vi "Main.vi"() -> ()   [LabVIEW 2014]
uses:
  <vilib>/addons/Fuzzy Logic/NI_Fuzzy_Logic_API.lvlib
  <vilib>/addons/Fuzzy Logic/FL Fuzzy Controller (MISO).vi
  <vilib>/express/express arith-compare/Formula/XNode/ExpressFormulaBlockNode.xnode
  <vilib>/express/express shared/transition.llb/Dynamic To Waveform Array.vi
  <vilib>/express/express arith-compare/Formula/Block/exnFormulaBlock how many pts in the wave.vi
  <vilib>/express/express shared/ex_Modify Signal Name.vi
  <vilib>/express/express shared/transition.llb/Waveform Array To Dynamic.vi
panel:
  out "Control History":dbl(graph)
  out "Sensors History":dynamicdata(graph)
  out "Error bar":string
  out "Information":string
  out "Danger":bool
  out "Status":string
  out "Thermistor III":dbl(slide) scale=0.0..100.0
  out "Thermistor II":dbl(slide) scale=0.0..100.0
  out "LM-35 II":dbl(slide) scale=0.0..100.0
  out "LM-35 III":dbl(slide) scale=0.0..100.0
  out "Thermistor I":dbl(slide) scale=0.0..100.0
  out "LM-35 I":dbl(slide) scale=0.0..100.0
  out "Final Control":dbl(knob) scale=0.0..1.0
  out "LM-35 Intel":dbl(knob) scale=0.0..10.0
  out "Thermistors Intel":dbl(knob) scale=0.0..10.0
  in  "Control System":bool
  # "In Celsius"
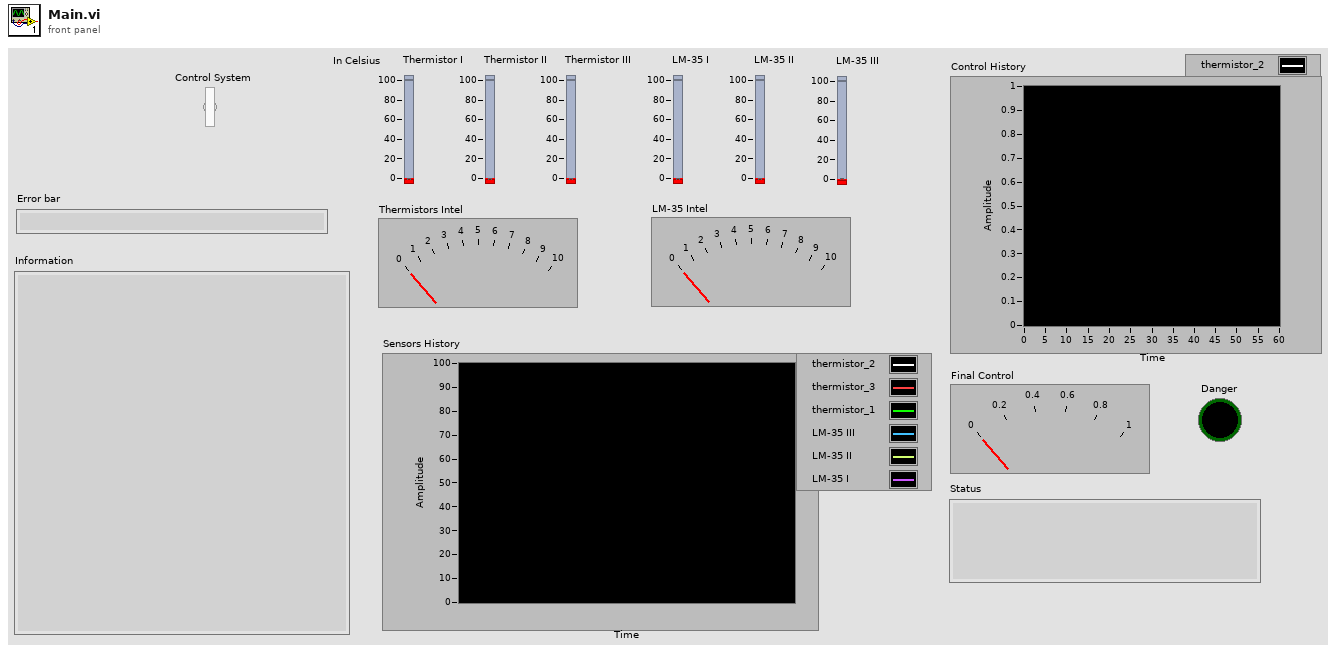
[diagram p1: front panel]
types:
  T1 = typedef "NI_Fuzzy_Logic_API.lvlib/FL System.ctl" = cluster{"input variables":T2[], "output variables":T2[], "rules":T5[], "defuzzification method":T11, "description":string, "user MF interpolating polynomials":T12[]}
  T2 = typedef "NI_Fuzzy_Logic_API.lvlib/FL Variable.ctl" = cluster{"name":string, "range":dbl[], "MFs":T3[]}
  T3 = typedef "NI_Fuzzy_Logic_API.lvlib/FL Membership Function.ctl" = cluster{"name":string, "shape":T4, "points":dbl[], "color":u32, "user-defined shape index":i32}
  T4 = typedef "NI_Fuzzy_Logic_API.lvlib/FL Membership Function Shape.ctl" = u16
  T5 = typedef "NI_Fuzzy_Logic_API.lvlib/FL Rule.ctl" = cluster{"antecedents":T6[], "antecedent connective":T8, "consequents":T9[], "consequent implication":T10, "degree of support":dbl}
  T6 = typedef "NI_Fuzzy_Logic_API.lvlib/FL Antecedent.ctl" = cluster{"Var Index":i32, "MF Index":i32, "Cond":T7}
  T7 = typedef "NI_Fuzzy_Logic_API.lvlib/FL Modifier.ctl" = u16
  T8 = typedef "NI_Fuzzy_Logic_API.lvlib/FL Antecedent Connective.ctl" = u16
  T9 = typedef "NI_Fuzzy_Logic_API.lvlib/FL Consequent.ctl" = cluster{"Var Index":i32, "MF Index":i32, "Cond":T7}
  T10 = typedef "NI_Fuzzy_Logic_API.lvlib/FL Consequent Implication.ctl" = u16
  T11 = typedef "NI_Fuzzy_Logic_API.lvlib/FL Defuzzification.ctl" = u16
  T12 = typedef "NI_Fuzzy_Logic_API.lvlib/FL Interpolating polynomials.ctl" = cluster{"X":dbl[], "Y":dbl[], "Y(x) coeff":dbl[][], "X(y) coeff":dbl[][], "Area(y) coeff":dbl[][], "coa_x(y) coeff":dbl[][]}
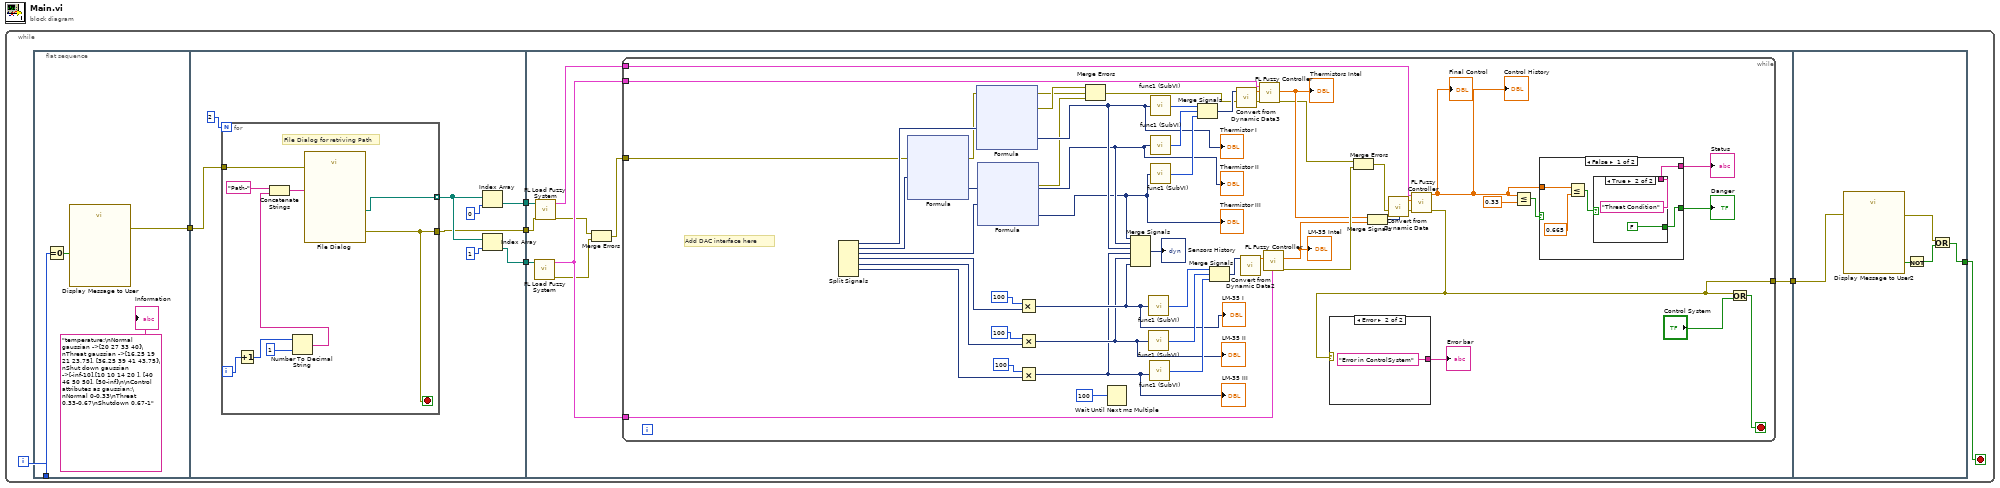
[diagram p0: block diagram]
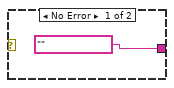
[diagram p2: hidden frame]
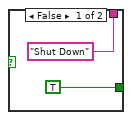
[diagram p3: hidden frame]
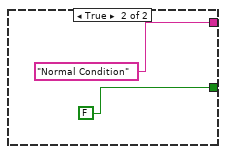
[diagram p4: hidden frame]
diagram:
  n1 = while {
    i -> [w7]
    stop <- w5 stop-if-true
    n2 = flat-sequence {
      tunnel: w7 -> [w10]
      tunnel: [w8] -> w4
      tunnel: w4 -> [w18]
      tunnel: [w14] -> w3
      tunnel: [w13] -> w2
      tunnel: [w12] -> w1
      tunnel: [w37] -> w6
      tunnel: w3 -> [w34]
      tunnel: w2 -> [w33]
      tunnel: w1 -> [w32]
      tunnel: [w519] -> w5
      tunnel: w6 -> [w522]
      frame #0 {
        n3 = Equal To 0?(x=w10) -> (x = 0?=w11:bool)
        n4 = call "Display Message to User"("Enable"=w11) -> ("error out"=w8:errorcluster)  [unwired: 9 in, 1 out]
        "Information" <- "temperature:\nNormal gaussian ->[20 27 33 40]\nThreat gaussian ->[16.25 19 21 23.75], [36.25 39 41 43.75]\nShut down gaussian ->[-inf-10],[10 10 14 20 ], [40 46 50 50], [50-inf]\n\nControl attributes as gaussian:\nNormal 0-0.33\nThreat 0.33-0.67\nShutdown 0.67-1" ("Information")
      }
      frame #1 {
        n5 = for {
          N: 2 -> [_]
          tunnel: [w28] -> w12
          tunnel: w18 -> [w21]
          tunnel: [w20] -> w15 mode=indexing
          i -> [w23]
          stop <- w28 stop-if-true
          # "File Dialog for retriving Path"
          n6 = Increment(x=w23) -> (x+1=w22:i32)
          n7 = Number To Decimal String(number=w22, width (-)=i16 1) -> (decimal integer string=w25:string)
          n8 = Concatenate Strings("Path-" ("string"), w25) -> (w27:string)
          n9 = call "File Dialog"("prompt"=w27, "error in"=w21) -> ("selected path"=w20:path, "error out"=w28:errorcluster)  [unwired: 10 in, 2 out]
        }
        n10 = Index Array(array=w15, index=1) -> (element=w13:path)
        n11 = Index Array(array=w15, index=0) -> (element=w14:path)
      }
      frame #2 {
        n12 = call <vilib>:"FL Load Fuzzy System.vi"("file path"=w33) -> ("error out"=w31:errorcluster, "fuzzy system out"=w35:T1)  [unwired: 9 in]
        n13 = call <vilib>:"FL Load Fuzzy System.vi"("error in (no error)"=w32, "file path"=w34) -> ("error out"=w30:errorcluster, "fuzzy system out"=w36:T1)  [unwired: 8 in]
        n14 = Merge Errors(w30, w31) -> (w29:errorcluster)
        n15 = while {
          tunnel: [w79] -> w37
          tunnel: w35 -> [w61]
          tunnel: w36 -> [w60]
          tunnel: w35 -> [w59]
          tunnel: w29 -> [w42]
          stop <- w84 stop-if-true
          # "Add DAC interface here"
          n16 = Split Signals() -> (w48:dynamicdata, w47:dynamicdata, w46:dynamicdata, w45:dynamicdata, w44:dynamicdata, w43:dynamicdata)  [unwired: 8 in, 1 out]
          n17 = xnode "Formula"("Voltage"=w47, "error in (no error)"=w42) -> ("Result"=w56:dynamicdata, "error out"=w39:errorcluster)
          "Thermistor II" <- w56
          n18 = xnode "Formula"("Voltage"=w48) -> ("Result"=w57:dynamicdata, "error out"=w40:errorcluster)  [unwired: 1 in]
          "Thermistor I" <- w57
          n19 = xnode "Formula"("Voltage"=w46) -> ("Result"=w55:dynamicdata, "error out"=w41:errorcluster)  [unwired: 1 in]
          "Thermistor III" <- w55
          n20 = Multiply(x=100, y=w45) -> (x*y=w54:dynamicdata)
          "LM-35 I" <- w54
          n21 = Multiply(x=100, y=w44) -> (x*y=w53:dynamicdata)
          "LM-35 II" <- w53
          n22 = Multiply(x=100, y=w43) -> (x*y=w52:dynamicdata)
          "LM-35 III" <- w52
          n23 = Merge Errors(w40, w39, w41) -> (w38:errorcluster)
          n24 = Wait Until Next ms Multiple(millisecond multiple=100) -> ()  [unwired: 1 out]
          n25 = Merge Signals(w55, w56, w57, w52, w53, w54) -> (→"Sensors History":dynamicdata)
          n26 = call "func1 (SubVI).vi"("input in"=w54) -> ("input out"=w74:i32)
          n27 = call "func1 (SubVI).vi"("input in"=w53) -> ("input out"=w73:i32)
          n28 = call "func1 (SubVI).vi"("input in"=w52) -> ("input out"=w72:i32)
          n29 = call "func1 (SubVI).vi"("input in"=w57) -> ("input out"=w62:i32)
          n30 = call "func1 (SubVI).vi"("input in"=w56) -> ("input out"=w63:i32)
          n31 = call "func1 (SubVI).vi"("input in"=w55) -> ("input out"=w64:i32)
          n32 = Merge Signals(w62, w63, w64) -> (w66:dynamicdata)
          n33 = Merge Signals(w74, w73, w72) -> (w71:dynamicdata)
          n34 = call "Convert from Dynamic Data3"("Dynamic Data Type"=w66) -> ("Array"=w65:dbl[])  [unwired: 3 in]
          n35 = call "Convert from Dynamic Data2"("Dynamic Data Type"=w71) -> ("Array"=w70:dbl[])  [unwired: 3 in]
          n36 = call-poly <vilib>:"FL Fuzzy Controller.vi"("error in (no error)"=w38, "input values"=w65, "fuzzy system in"=w61) -> ("error out"=w67:errorcluster, "output value"=w68:dbl)  [unwired: 4 in, 3 out]
          "Thermistors Intel" <- w68
          n37 = call-poly <vilib>:"FL Fuzzy Controller.vi"("input values"=w70, "fuzzy system in"=w59) -> ("error out"=w75:errorcluster, "output value"=w69:dbl)  [unwired: 5 in, 3 out]
          "LM-35 Intel" <- w69
          n38 = Merge Errors(w67, w75) -> (w78:errorcluster)
          n39 = Merge Signals(w68, w69) -> (w77:dynamicdata)
          n40 = call "Convert from Dynamic Data"("Dynamic Data Type"=w77) -> ("Array"=w76:dbl[])  [unwired: 3 in]
          n41 = call-poly <vilib>:"FL Fuzzy Controller.vi"("error in (no error)"=w78, "input values"=w76, "fuzzy system in"=w60) -> ("error out"=w79:errorcluster, "output value"=w80:dbl)  [unwired: 4 in, 3 out]
          "Final Control" <- w80
          "Control History" <- w80
          n42 = case shown="Error" w79 {
            tunnel: ["" "Error in ControlSystem"] -> w83
            frame No Error {
            }
            frame Error {
            }
          }
          "Error bar" <- w83
          n43 = Less Or Equal?(x=w80, y=0.33) -> (x <= y?=w86:bool)
          n44 = case shown="False" w86 {
            tunnel: w80 -> [w512 _]
            tunnel: [w509 "Normal Condition"] -> w85
            tunnel: [w508 FALSE] -> w58
            frame False {
              n45 = Less Or Equal?(x=w512, y=0.665) -> (x <= y?=w510:bool)
              n46 = case shown="True" w510 {
                tunnel: ["Shut Down" "Threat Condition"] -> w509
                tunnel: [TRUE FALSE] -> w508
                frame False {
                }
                frame True {
                }
              }
            }
            frame True {
            }
          }
          "Status" <- w85
          "Danger" <- w58
          n47 = Or(x=w79, y="Control System") -> (x .or. y?=w84:bool)
        }
      }
      frame #3 {
        n48 = call "Display Message to User2"("error in (no error)"=w522) -> ("error out"=w520:errorcluster, "OK"=w523:bool)  [unwired: 9 in]
        n49 = Not(x=w523) -> (.not. x?=w521:bool)
        n50 = Or(x=w520, y=w521) -> (x .or. y?=w519:bool)
      }
    }
  }
